vi "Mouse Down_ RightClick cache.vi"(5 "Coords":T1, 7 "PlatMods":T2, 8 "error in (no error)":errorcluster, 10 "Refs":T13, 11 "Loop data in":T3={"TitleCollapse"=refnum, "MouseDownState"=enum."Idle", "RightClickCache"={"Mod"={"Ctrl"=FALSE, "Shift"=FALSE}, "CoordsStart"={"Horizontal"=0, "Vertical"=0}, "CoordsEnd"={"Horizontal"=0, "Vertical"=0}, "PlotAreaBounds"={"Left"=10, "Top"=10, "Right"=0, "Bottom"=0}, "slice"=[]}, "ZoomCache"={"SuppressedPlots"=[], "LeftAxis"={"NeedsRevert?"=FALSE, "Scale Fit"=0, "Range"={"Minimum"=0.0, "Maximum"=0.0, "Increment"=0.0, "Minor Increment"=0.0, "Start"=0.0}}, "RightAxis"={"NeedsRevert?"=FALSE, "Scale Fit"=0, "Range"={"Minimum"=0.0, "Maximum"=0.0, "Increment"=0.0, "Minor Increment"=0.0, "Start"=0.0}}, "Mod"={"Shift"=FALSE}}, "UpdateTime"=0.0, "keyboard"=refnum, "visible?"=FALSE}) -> (0 "error out":errorcluster, 3 "Loop data out":T3={"TitleCollapse"=refnum, "MouseDownState"=enum."Idle", "RightClickCache"={"Mod"={"Ctrl"=FALSE, "Shift"=FALSE}, "CoordsStart"={"Horizontal"=0, "Vertical"=0}, "CoordsEnd"={"Horizontal"=0, "Vertical"=0}, "PlotAreaBounds"={"Left"=10, "Top"=10, "Right"=0, "Bottom"=0}, "slice"=[]}, "ZoomCache"={"SuppressedPlots"=[], "LeftAxis"={"NeedsRevert?"=FALSE, "Scale Fit"=0, "Range"={"Minimum"=0.0, "Maximum"=0.0, "Increment"=0.0, "Minor Increment"=0.0, "Start"=0.0}}, "RightAxis"={"NeedsRevert?"=FALSE, "Scale Fit"=0, "Range"={"Minimum"=0.0, "Maximum"=0.0, "Increment"=0.0, "Minor Increment"=0.0, "Start"=0.0}}, "Mod"={"Shift"=FALSE}}, "UpdateTime"=0.0, "keyboard"=refnum, "visible?"=FALSE})   [LabVIEW 2021, in "RocketPlot.lvlib"]
uses:
  RocketPlot.lvlib
  TypeDefs/Plot UI references.ctl
  Classes/RocketPlotHandle/RocketPlotHandle.lvclass
  <userlib>/bjustice/TipStripOOPanel/Classes/TipPanelHandle/TipPanelHandle.lvclass
  TypeDefs/Plot top row.ctl
  TypeDefs/plot while loop data.ctl
  CollapsePanel/CollapsePanel.lvclass
  TypeDefs/MouseDownState.ctl
  TypeDefs/RightClickCache.ctl
  TypeDefs/RightClickCache PlatMod.ctl
  <vilib>/Utility/miscctls.llb/LVPoint32TypeDef.ctl
  <vilib>/Utility/miscctls.llb/LVRectTypeDef.ctl
  TypeDefs/Slice average.ctl
  TypeDefs/ZoomCache.ctl
  TypeDefs/RangeCache.ctl
  <vilib>/Utility/miscctls.llb/LVRangeTypeDef.ctl
  TypeDefs/ZoomCache PlatMod.ctl
  Draw PlotImageFront.vi
  RightClickUpdate.vi
  RightClickType.vi
  RightClickUpdate Delta.vi
  RightClickUpdate SliveAvg.vi
  Plot Load maker V2 - scaleread grid colors.vi
  Classes/TipTablePanel/new cell.vi
  Plot scale refnum to LUT name.vi
  Classes/TipTablePanel/TipTablePanel.lvclass
  C:/Program Files/National Instruments/LabVIEW 2021/user.lib/bjustice/TipStripOOPanel/Classes/TipPanel/TipPanel.lvclass
  Draw SliveAvg line.vi
  Draw Indentify line.vi
  Draw Delta Values line.vi
  <userlib>/bjustice/TipStripOOPanel/Classes/TipPanelHandle/TipStrip API.vi
  <userlib>/bjustice/TipStripOOPanel/Classes/TipPanelHandle/CMD - hide.vi
  Classes/TipTablePanel/New TipTable.vi
  <userlib>/bjustice/TipStripOOPanel/Classes/TipPanelHandle/CMD - show panel.vi
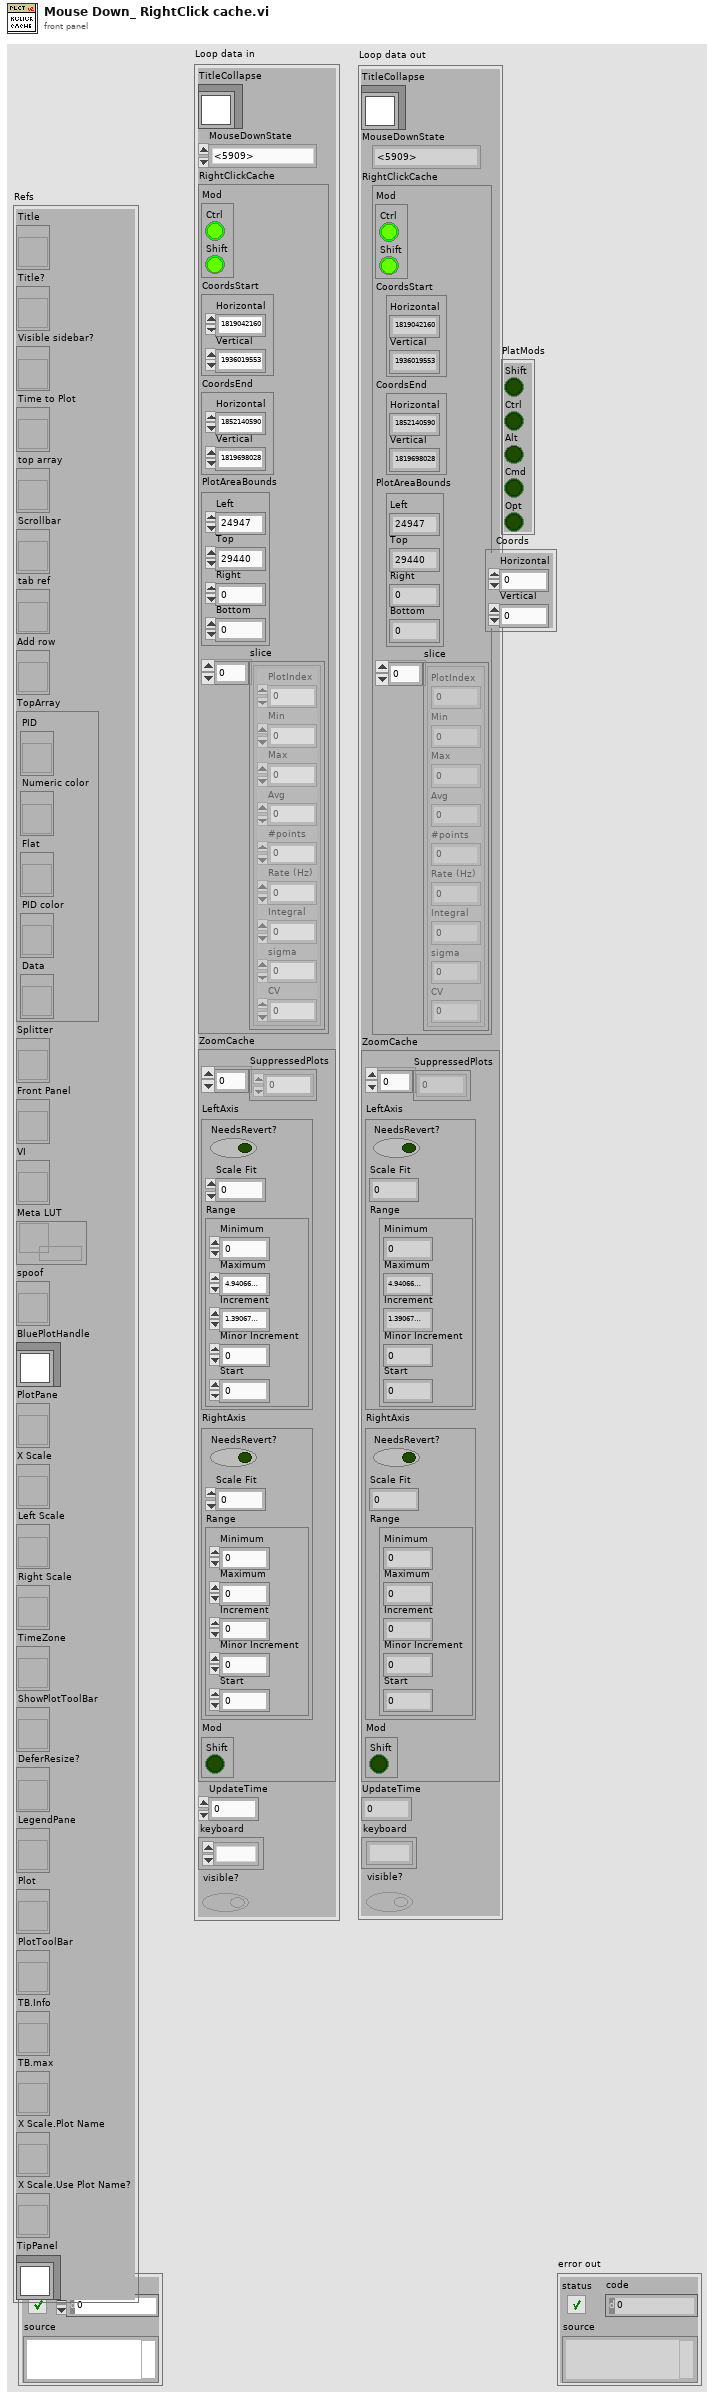
[diagram p1: front panel]
types:
  T1 = typedef "LVPoint32TypeDef.ctl" = cluster{"Horizontal":i32, "Vertical":i32}
  T2 = cluster{"Shift":bool, "Ctrl":bool, "Alt":bool, "Cmd":bool, "Opt":bool}
  T3 = typedef "RocketPlot.lvlib/plot while loop data.ctl" = cluster{"TitleCollapse":refnum<class "CollapsePanel.lvclass">, "MouseDownState":T4, "RightClickCache":T5, "ZoomCache":T9, "UpdateTime":dbl, "keyboard":refnum<k1>, "visible?":bool}
  T4 = typedef "RocketPlot.lvlib/MouseDownState.ctl" = enum16{"Idle", "Pan", "Zoom", "Zoom-Post", "RightClick"}
  T5 = typedef "RocketPlot.lvlib/RightClickCache.ctl" = cluster{"Mod":T6, "CoordsStart":T1, "CoordsEnd":T1, "PlotAreaBounds":T7, "slice":T8[]}
  T6 = typedef "RocketPlot.lvlib/RightClickCache PlatMod.ctl" = cluster{"Ctrl":bool, "Shift":bool}
  T7 = typedef "LVRectTypeDef.ctl" = cluster{"Left":i16, "Top":i16, "Right":i16, "Bottom":i16}
  T8 = typedef "RocketPlot.lvlib/Slice average.ctl" = cluster{"PlotIndex":i32, "Min":dbl, "Max":dbl, "Avg":dbl, "#points":u32, "Rate (Hz)":dbl, "Integral":dbl, "sigma":dbl, "CV":dbl}
  T9 = typedef "RocketPlot.lvlib/ZoomCache.ctl" = cluster{"SuppressedPlots":i32[], "LeftAxis":T10, "RightAxis":T10, "Mod":T12}
  T10 = typedef "RocketPlot.lvlib/RangeCache.ctl" = cluster{"NeedsRevert?":bool, "Scale Fit":u8, "Range":T11}
  T11 = typedef "LVRangeTypeDef.ctl" = cluster{"Minimum":dbl, "Maximum":dbl, "Increment":dbl, "Minor Increment":dbl, "Start":dbl}
  T12 = typedef "RocketPlot.lvlib/ZoomCache PlatMod.ctl" = cluster{"Shift":bool}
  T13 = typedef "RocketPlot.lvlib/Plot UI references.ctl" = cluster{"Title":refnum<vi>, "Title?":refnum<vi>, "Visible sidebar?":refnum<vi>, "Time to Plot":refnum<vi>, "top array":refnum<vi>, "Scrollbar":refnum<vi>, "tab ref":refnum<vi>, "Add row":refnum<vi>, "TopArray":cluster{"PID":refnum<vi>, "Numeric color":refnum<vi>, "Flat":refnum<vi>, "PID color":refnum<vi>, "Data":refnum<vi>}, "Splitter":refnum<vi>, "Front Panel":refnum<vi>, "VI":refnum<vi>, "Meta LUT":refnum<data-value>, "spoof":refnum<vi>, "BluePlotHandle":refnum<class "RocketPlotHandle.lvclass">, "PlotPane":refnum<vi>, "X Scale":refnum<vi>, "Left Scale":refnum<vi>, "Right Scale":refnum<vi>, "TimeZone":refnum<vi>, "ShowPlotToolBar":refnum<vi>, "DeferResize?":refnum<vi>, "LegendPane":refnum<vi>, "Plot":refnum<vi>, "PlotToolBar":refnum<vi>, "TB.Info":refnum<vi>, "TB.max":refnum<vi>, "X Scale.Plot Name":refnum<vi>, "X Scale.Use Plot Name?":refnum<vi>, "TipPanel":refnum<class "TipPanelHandle.lvclass">}
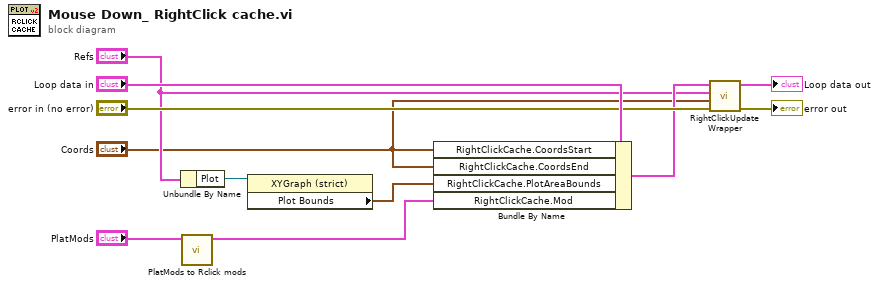
[diagram p0: block diagram]
diagram:
  n1 = Unbundle By Name("Refs") -> ("Plot"=w10:refnum<vi>)
  n2 = call "PlatMods to Rclick mods.vi"("PlatMods"="PlatMods") -> ("Rclick mods"=w7:T6)  [unwired: 10 in]
  n3 = property on="Property Node" class="XYGraph (strict)"(reference=w10) -> ("Plot Bounds"=w9:T7)  [unwired: 1 in, 2 out]
  n4 = Bundle By Name(cluster="Loop data in", "RightClickCache.CoordsStart"="Coords", "RightClickCache.CoordsEnd"="Coords", "RightClickCache.PlotAreaBounds"=w9, "RightClickCache.Mod"=w7) -> (w4:T3)
  n5 = call "RightClickUpdate Wrapper.vi"("error in (no error)"="error in (no error)", "Coords (no change)"="Coords", "Refs"="Refs", "Loop data in"=w4) -> ("error out"=→"error out":errorcluster, "Loop data out"=→"Loop data out":T3)  [unwired: 6 in]
